vi "Calc Time and Rate to Gallons.vi"(0 "Elapsed Time(s)":dbl, 1 "Previous Rate":dbl, 2 "Current Rate":dbl) -> (15 "Gallons":dbl)   [LabVIEW 2009]
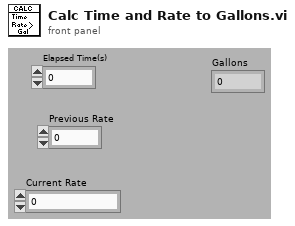
[diagram p1: front panel]
types:
  T1 = enum16{"Method1", "Method2", "Method3", "Method4"}
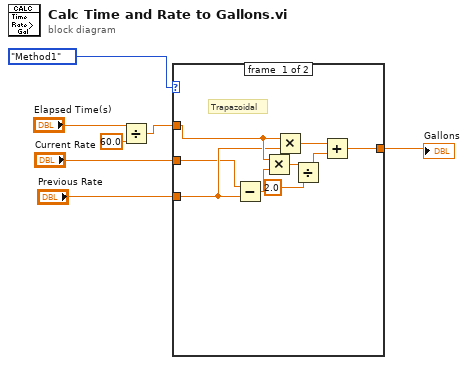
[diagram p0: block diagram]
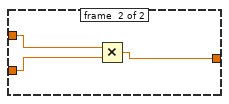
[diagram p2: hidden frame]
diagram:
  n1 = Divide(x="Elapsed Time(s)", y=60.0) -> (x/y=w2:dbl)
  n2 = case shown="\"Method1\", Default" T1."Method1" {
    tunnel: w2 -> [w11 w18]
    tunnel: "Previous Rate" -> [w10 _]
    tunnel: "Current Rate" -> [w9 w19]
    tunnel: [w8 w17] -> w4
    frame #0 {
      # "Trapazoidal"
      n3 = Subtract(x=w9, y=w10) -> (x-y=w16:dbl)
      n4 = Multiply(x=w11, y=w16) -> (x*y=w13:dbl)
      n5 = Multiply(x=w11, y=w10) -> (x*y=w12:dbl)
      n6 = Divide(x=w13, y=2.0) -> (x/y=w14:dbl)
      n7 = Add(x=w12, y=w14) -> (x+y=w8:dbl)
    }
    frame #1 {
      n8 = Multiply(x=w18, y=w19) -> (x*y=w17:dbl)
    }
  }
  "Gallons" <- w4
